vi "SetupContinuosAcquisition.vi"(8 "error in (no error)":errorcluster, 11 "CameraSession in":refnum<class "CS250-CameraHardwareClass.lvclass">) -> (0 "error out":errorcluster, 3 "CameraSession out":refnum<class "CS250-CameraHardwareClass.lvclass">)   [LabVIEW 2013, in "CS250-CameraHardwareClass.lvclass"]
doc: "Setup the continuos acquisition session"
uses:
  CS250-CameraHardwareClass.lvclass
  CS250-CameraHardwareClass.lvclass/CS250-CameraHardwareClass.ctl
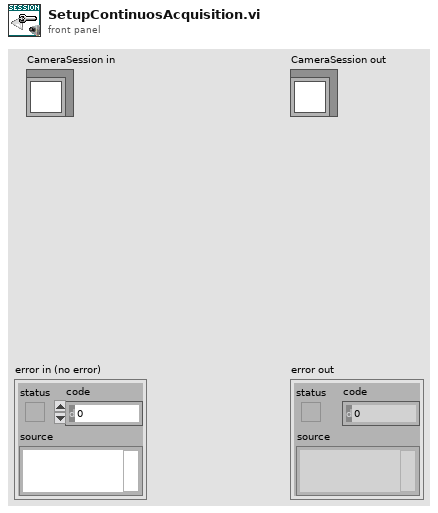
[diagram p1: front panel]
types:
  T1 = typedef "CamCluster.ctl" = cluster{"hcam out":i16, "TempImage":T2, "Pointer":u32, "exp_bytes out":u32, "rgn_array":cluster{"s1":u16, "s2":u16, "sbin":u16, "p1":u16, "p2":u16, "pbin":u16}, "CameraName":string}
  T2 = typedef "IMAQ Image.ctl" = refnum<image>
  T3 = typedef "TriggerMode_TypDef.ctl" = enum16{"Timed", "Strobed", "Bulb", "Trigger first", "Flash", "Variable Timed"}
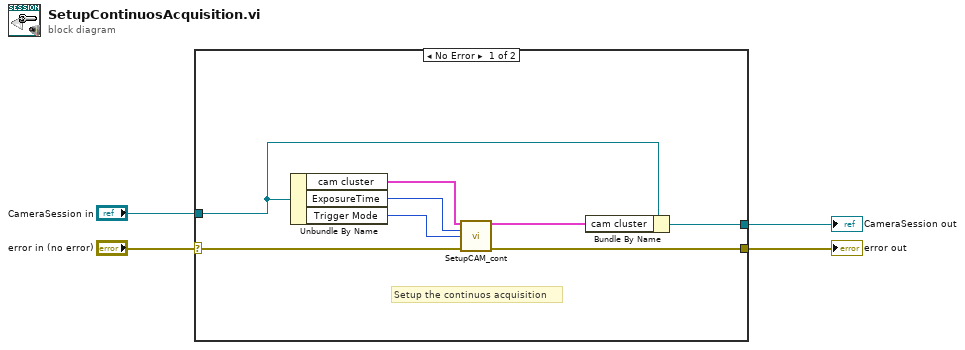
[diagram p0: block diagram]
diagram:
  n1 = case shown="No Error" "error in (no error)" {
    selector: "error in (no error)" -> [w12 w14]
    tunnel: [w11 w14] -> w3
    tunnel: [w10 w13] -> w1
    tunnel: "CameraSession in" -> [w7 w13]
    frame No Error {
      # "Setup the continuos acquisition"
      n2 = Unbundle By Name(w7) -> ("cam cluster"=w8:T1, "ExposureTime"=w6:u32, "Trigger Mode"=w5:T3)
      n3 = call "SetupCAM_cont.vi"("Cam cluster in"=w8, "exposure_time"=w6, "trigger mode (input)"=w5, "error in (no error)"=w12) -> ("cam cluster out"=w9:T1, "error out"=w11:errorcluster)  [unwired: 10 in]
      n4 = Bundle By Name(cluster=w7, "cam cluster"=w9) -> (w10:refnum<class "CS250-CameraHardwareClass.lvclass">)
    }
    frame Error {
    }
  }
  "error out" <- w3
  "CameraSession out" <- w1
